vi "Save_Info.vi"(8 "error in (no error)":errorcluster, 11 "AB_RESTfulWebService in":refnum<class "AB_RESTfulWebService.lvclass">) -> (0 "error out":errorcluster, 3 "AB_RESTfulWebService out":refnum<class "AB_RESTfulWebService.lvclass">)   [LabVIEW 2020, in "AB_RESTfulWebService.lvclass"]
uses:
  <vilib>/AppBuilder/AB_Classes/RESTful/AB_RESTfulWebService.lvclass
  e:/builds/penguin/labview/branches/2020/dev/dist/vi.lib/AppBuilder/AB_Classes/Build/AB_Build.lvclass
  <vilib>/AppBuilder/RW_Project/AB_RW_Project_RESTfulWebService_Data.ctl
  <vilib>/AppBuilder/RW_Project/AB_RW_Project_RESTful_RoutingTemplate.ctl
  <vilib>/AppBuilder/AB_Classes/RESTful/AB_RESTful_RoutingType.ctl
  <vilib>/AppBuilder/AB_Classes/RESTful/AB_RESTful_HTTPMethodType.ctl
  <vilib>/AppBuilder/RW_Project/AB_RW_Project_PropBag_Action.ctl
  <vilib>/AppBuilder/AB_Classes/RESTful/AB_RESTfulWebService.lvclass/AB_RESTfulWebService.ctl
  <vilib>/Utility/error.llb/whitespace.ctl
  <vilib>/AppBuilder/AB_Classes/WebService/AB_WebService.lvclass
  <vilib>/AppBuilder/AB_Classes/Build/AB_Build.lvclass
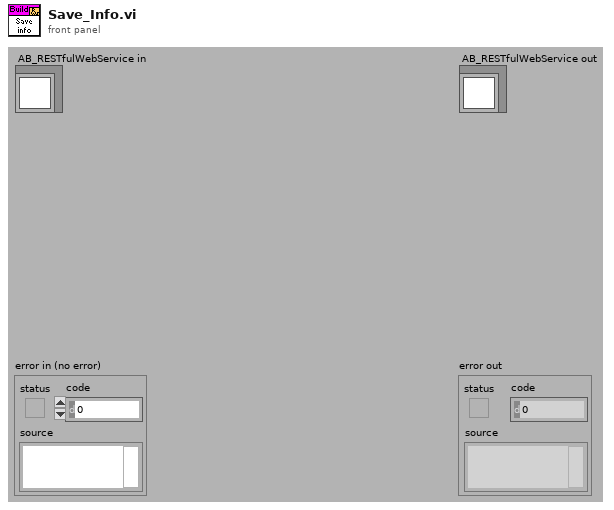
[diagram p1: front panel]
types:
  T1 = typedef "AB_RW_Project_RESTfulWebService_Data.ctl" = cluster{"routing templates":T2[], "defaultStaticDoc":string}
  T2 = typedef "AB_RW_Project_RESTful_RoutingTemplate.ctl" = cluster{"Template":string, "Routing Type":T3, "HTTP Method Type":T4, "VIName":string, "Default String":string, "Require API key":bool, "Auth permissions":string}
  T3 = typedef "AB_RESTful_RoutingType.ctl" = enum32{"Method", "Static"}
  T4 = typedef "AB_RESTful_HTTPMethodType.ctl" = enum32{"GET", "POST", "PUT", "DELETE"}
  T5 = typedef "AB_RW_Project_PropBag_Action.ctl" = enum16{"read", "write", "clear", "readPrevious", "writePrevious", "clearPrevious"}
  T6 = typedef "AB_RESTfulWebService.ctl" = cluster{"routing templates":T7[], "defaultStaticDoc":string, "eng_attributes":T8[], "Privilege Mapping":cluster{"Privilege":string, "Description":string, "Role":string}[]}
  T7 = typedef "AB_RESTful_RoutingTemplate.ctl" = cluster{"Template":string, "Routing Type":T3, "HTTP Method Type":T4, "VIName":string, "Default String":string, "Require API key":bool, "Auth permissions":string[], "eng_Static Alias":string, "Required Privilege":string}
  T8 = typedef "AB_RESTful_ServiceAttribute.ctl" = cluster{"Name":string, "Service Attribute Type":T9, "Value":string}
  T9 = typedef "AB_RESTful_ServiceAttributeType.ctl" = enum32{"String", "Path"}
  T10 = typedef "whitespace.ctl" = u16
  T11 = typedef "AB_Build.ctl" = cluster{"buildSpecName":string, "buildSpecDescription":string, "destinations":refnum<class "AB_Destination.lvclass">[], "exclusionOption":T12, "defaultLanguage":string, "supportedLanguages":string[], "excludedDirectories":path[], "buildContext":refnum<vi>, "buildObject":T13, "preview":bool, "programatic":bool, "progressBarEvents":T14, "userLog_Path":path, "preActionID":string, "preAction_Path":path, "postActionID":string, "postAction_Path":path, "eng_checkForBrokenVIs?":bool, "eng_verboseLinkerErrors?":bool, "localDest_Path":path, "targetDest_Path":path, "removeVIObject":u16, "cache":refnum<class "PreviewCache.lvclass">, "use cache":bool, "previewCache_ID":string, "buildCache_ID":string, "eng_TempLocalDest_Path":path, "eng_collectDependencies?":bool, "versionInfo":cluster{"buildVersion":cluster{"major":u16, "minor":u16, "patch":u16, "build":u16}, "autoIncrement":bool}, "eng_enableVIChecksums":bool}
  T12 = typedef "AB_Exclusion_Option.ctl" = cluster{"typedefs":bool, "polymorphicVIs":bool, "unusedLibraryItems":bool, "modifyLibraryFile":bool, "edit-timeDependencies":bool, "inlineVIs":bool, "dependent PPLs":bool, "dependent DLLs":bool}
  T13 = typedef "ItemRef.ctl" = u64
  T14 = typedef "provcom_ProgressBar_Events.ctl" = cluster{"newJob":refnum<user-event>, "newItem":refnum<user-event>, "errorMsg":T15, "cancel":refnum<user-event>}
  T15 = typedef "mxLvBuildError.ctl" = refnum<user-event>
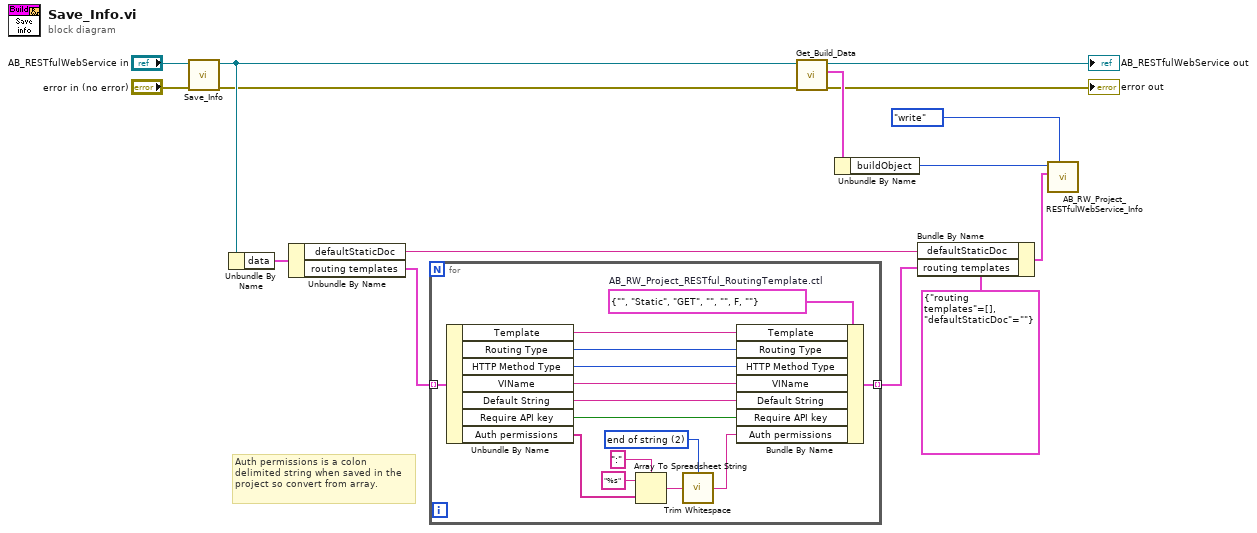
[diagram p0: block diagram]
diagram:
  # "Auth permissions is a colon delimited string when saved in the project so convert from array."
  n1 = call-parent "Save_Info.vi"("error in (no error)"="error in (no error)", "AB_WebService in"="AB_RESTfulWebService in") -> ("error out"=w10:errorcluster, "AB_WebService out"=w11:refnum<class "AB_RESTfulWebService.lvclass">)  [unwired: 8 in]
  n2 = Unbundle By Name(w11) -> ("data"=w5:T6)
  n3 = Unbundle By Name(w5) -> ("defaultStaticDoc"=w4:string, "routing templates"=w3:T7[])
  n4 = for {
    tunnel: w3 -> [w30] mode=indexing
    tunnel: [w22] -> w2 mode=indexing
    w18 = T10 2 items=["both", "start of string", "end of string"] ("location (both)")
    w29 = T2 {"Template"="", "Routing Type"=enum."Static", "HTTP Method Type"=enum."GET", "VIName"="", "Default String"="", "Require API key"=FALSE, "Auth permissions"=""}  # AB_RW_Project_RESTful_RoutingTemplate.ctl
    n5 = Unbundle By Name(w30) -> ("Template"=w28:string, "Routing Type"=w27:T3, "HTTP Method Type"=w26:T4, "VIName"=w25:string, "Default String"=w24:string, "Require API key"=w23:bool, "Auth permissions"=w16:string[])
    n6 = Array To Spreadsheet String(delimiter (Tab)=":", array=w16, 3:"%s" ("format string")) -> (spreadsheet string=w19:string)
    n7 = call <vilib>:"Trim Whitespace.vi"("string"=w19, "location (both)"=w18) -> ("trimmed string"=w17:string)
    n8 = Bundle By Name(cluster=w29, "Template"=w28, "Routing Type"=w27, "HTTP Method Type"=w26, "VIName"=w25, "Default String"=w24, "Require API key"=w23, "Auth permissions"=w17) -> (w22:T2)
  }
  n9 = call <vilib>:"Get_Build_Data.vi"("error in (no error)"=w10, "Class in"=w11) -> ("error out"=→"error out":errorcluster, "data"=w13:T11, "Class out"=→"AB_RESTfulWebService out":refnum<class "AB_RESTfulWebService.lvclass">)  [unwired: 7 in]
  n10 = Unbundle By Name(w13) -> ("buildObject"=w1:T13)
  n11 = Bundle By Name(cluster=T1 {"routing templates"=[], "defaultStaticDoc"=""} ("RESTfulWebServiceInfo in"), "defaultStaticDoc"=w4, "routing templates"=w2) -> (w6:T1)
  n12 = call <vilib>:"AB_RW_Project_RESTfulWebService_Info.vi"("action"=AB_RW_Project_PropBag_Action."write", "RESTfulWebServiceInfo in"=w6, "Object In"=w1) -> ()  [unwired: 6 in, 3 out]
